vi "Viewport Size Separator.vi"(8 "error in (no error)":errorcluster, 10 "Boolean":bool, 11 "MxdSgG in":refnum<class "MixedSignalGraph.lvclass">) -> (0 "error out":errorcluster, 3 "MxdSgG out":refnum<class "MixedSignalGraph.lvclass">)   [LabVIEW 2023, in "MixedSignalGraph.lvclass"]
uses:
  MixedSignalGraph.lvclass
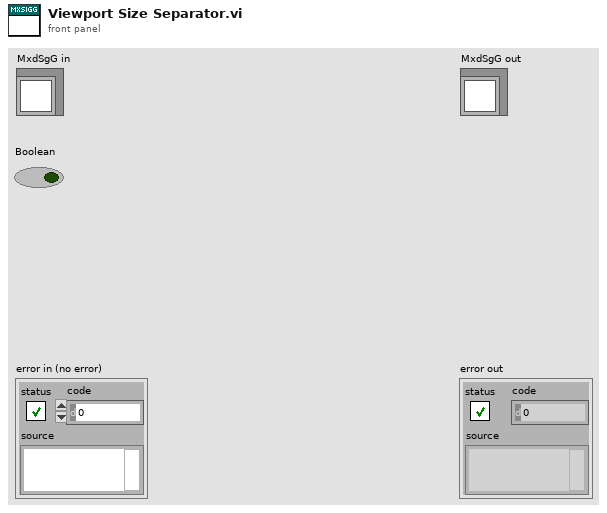
[diagram p1: front panel]
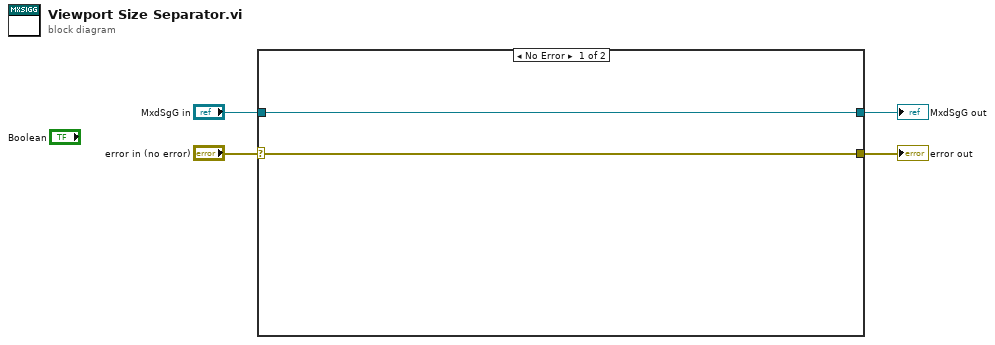
[diagram p0: block diagram]
diagram:
  n1 = case shown="No Error" "error in (no error)" {
    selector: "error in (no error)" -> [w5 w8]
    tunnel: [w5 w8] -> w3
    tunnel: [w6 w7] -> w1
    tunnel: "MxdSgG in" -> [w6 w7]
    frame No Error {
    }
    frame Error {
    }
  }
  "error out" <- w3
  "MxdSgG out" <- w1
